vi "Push Border.vi"(8 "1D Maze":i32[](array[numeric]), 9 "Post":T1, 11 "Class":refnum<class "Pinwheel.lvclass">) -> (3 "Class":refnum<class "Pinwheel.lvclass">)   [LabVIEW 2015, in "Pinwheel.lvclass"]
uses:
  Pinwheel.lvclass
  Square/Square.lvclass
  Type Defs/Direction Enum.ctl
  Type Defs/SB Type Defs.lvlib
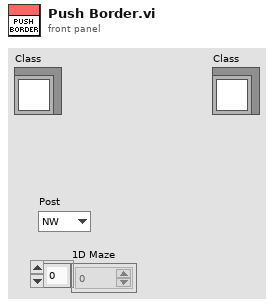
[diagram p1: front panel]
types:
  T1 = typedef "SB Type Defs.lvlib/Direction Enum.ctl" = enum16{"NW", "N", "NE", "E", "SE", "S", "SW", "W"}
  T2 = typedef "Pinwheel.lvclass/DVR Cluster.ctl" = cluster{"N":i32, "E":i32, "S":i32, "W":i32, "OD":T1, "NR":i32, "ER":i32, "SR":i32, "WR":i32, "NE":i32, "EE":i32, "SE":i32, "WE":i32, "Team":i32}
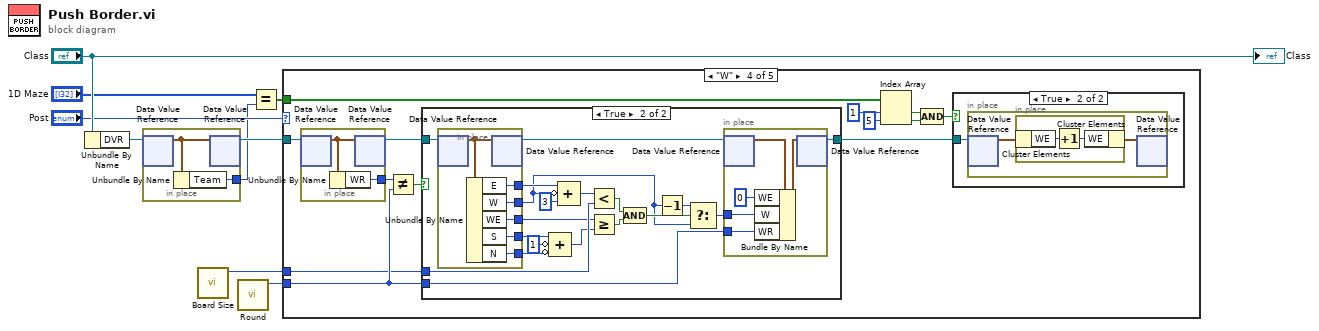
[diagram p0: block diagram]
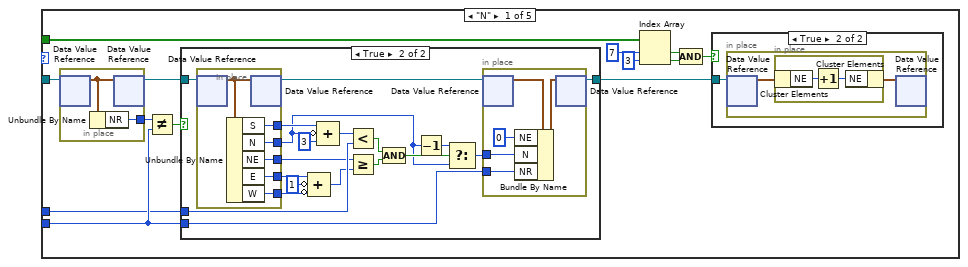
[diagram p2: hidden frame]
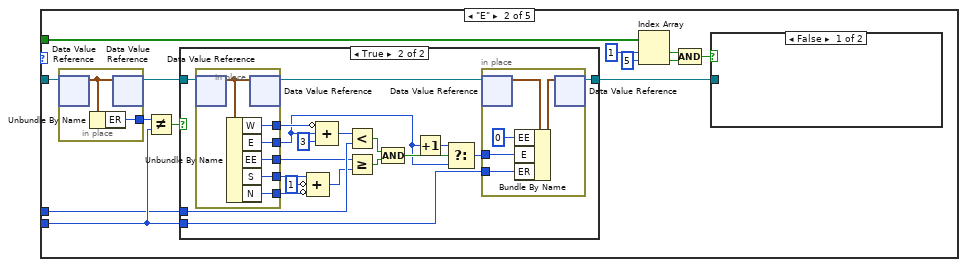
[diagram p5: hidden frame]
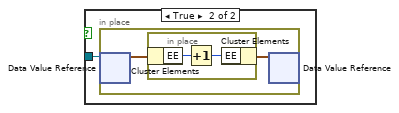
[diagram p7: hidden frame]
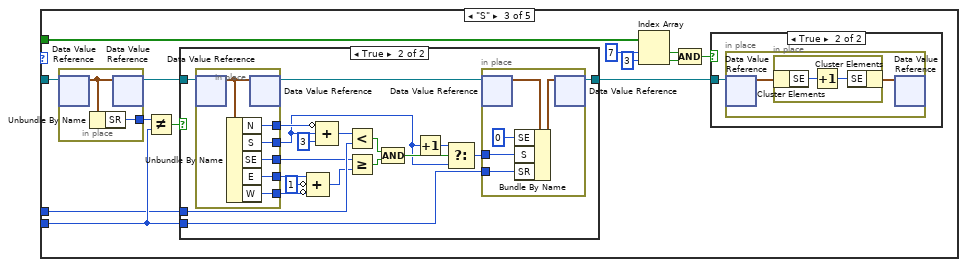
[diagram p8: hidden frame]
diagram:
  n1 = Unbundle By Name("Class") -> ("DVR"=w5:refnum<data-value>)
  n2 = in-place {
    in-place-border: [w10] -> w3
    n3 = in-place-dvr #1(w5) -> (w11:T2)  [unwired: 1 out]
    n4 = Unbundle By Name(w11) -> ("Team"=w10:i32)
    n5 = in-place-dvr #1(w11) -> (w4:refnum<data-value>)  [unwired: 1 out]
  }
  n6 = call "Board Size.vi"() -> ("Board Size"=w6:i32)  [unwired: 11 in]
  n7 = call "Round.vi"() -> ("Round"=w7:i32)  [unwired: 11 in]
  n8 = Equal?(x="1D Maze", y=w3) -> (x = y?=w1:bool[])
  n9 = case shown="\"W\"" "Post" {
    tunnel: w4 -> [w18 w69 w120 w171 _]
    tunnel: w1 -> [w24 w75 w126 w177 _]
    tunnel: w7 -> [w14 w65 w116 w167 _]
    tunnel: w6 -> [w13 w64 w115 w166 _]
    frame "N" {
      n10 = in-place {
        in-place-border: [w56] -> w17
        n11 = in-place-dvr #2(w18) -> (w57:T2)  [unwired: 1 out]
        n12 = Unbundle By Name(w57) -> ("NR"=w56:i32)
        n13 = in-place-dvr #2(w57) -> (w16:refnum<data-value>)  [unwired: 1 out]
      }
      n14 = Not Equal?(x=w17, y=w14) -> (x != y?=w15:bool)
      n15 = case shown="True" w15 {
        tunnel: w16 -> [w25 w43]
        tunnel: w14 -> [_ w44]
        tunnel: w13 -> [_ w37]
        tunnel: [w25 w32] -> w12
        frame False {
        }
        frame True {
          n16 = in-place {
            in-place-border: [w49] -> w28
            in-place-border: [w48] -> w34
            in-place-border: [w47] -> w40
            in-place-border: [w46] -> w31
            in-place-border: [w45] -> w30
            n17 = in-place-dvr #3(w43) -> (w50:T2)  [unwired: 1 out]
            n18 = Unbundle By Name(w50) -> ("S"=w47:i32, "N"=w48:i32, "NE"=w49:i32, "E"=w46:i32, "W"=w45:i32)
            n19 = in-place-dvr #3(w50) -> (w42:refnum<data-value>)  [unwired: 1 out]
          }
          n20 = Compound Arithmetic op=ADD(w31, invert 1 ("value"), invert w30) -> (w27:i32)
          n21 = Compound Arithmetic op=ADD(w40, invert w34, 3 ("value")) -> (w38:i32)
          n22 = Less?(x=w38, y=w37) -> (x < y?=w36:bool)
          n23 = Greater Or Equal?(x=w28, y=w27) -> (x >= y?=w29:bool)
          n24 = Compound Arithmetic op=AND(w36, w29) -> (w41:bool)
          n25 = Decrement(x=w34) -> (x-1=w35:i32)
          n26 = Select(t=w35, s=w41, f=w34) -> (s? t:f=w33:i32)
          n27 = in-place {
            in-place-border: w44 -> [w52]
            in-place-border: w33 -> [w53]
            n28 = in-place-dvr #4(w42) -> (w55:T2)  [unwired: 1 out]
            n29 = Bundle By Name(cluster=w55, "NE"=0, "N"=w53, "NR"=w52) -> (w54:T2)
            n30 = in-place-dvr #4(w54) -> (w32:refnum<data-value>)  [unwired: 1 out]
          }
        }
      }
      n31 = Index Array(array=w24, index #1=7 ("index"), index #2=3 ("index")) -> (element #1=w21:bool, element #2=w20:bool)
      n32 = Compound Arithmetic op=AND(w21, w20) -> (w19:bool)
      n33 = case shown="True" w19 {
        tunnel: w12 -> [_ w58]
        frame False {
        }
        frame True {
          n34 = in-place {
            n35 = in-place-dvr #5(w58) -> (w60:T2)  [unwired: 1 out]
            n36 = in-place {
              n37 = in-place-cluster #6(w60) -> ("NE"=w62:i32)
              n38 = Increment(x=w62) -> (x+1=w61:i32)
              n39 = in-place-cluster #6("NE"=w61) -> (w59:T2)
            }
            n40 = in-place-dvr #5(w59) -> ()  [unwired: 2 out]
          }
        }
      }
    }
    frame "E" {
      n41 = in-place {
        in-place-border: [w107] -> w68
        n42 = in-place-dvr #7(w69) -> (w108:T2)  [unwired: 1 out]
        n43 = Unbundle By Name(w108) -> ("ER"=w107:i32)
        n44 = in-place-dvr #7(w108) -> (w67:refnum<data-value>)  [unwired: 1 out]
      }
      n45 = Not Equal?(x=w68, y=w65) -> (x != y?=w66:bool)
      n46 = case shown="True" w66 {
        tunnel: w67 -> [w76 w94]
        tunnel: w65 -> [_ w95]
        tunnel: w64 -> [_ w88]
        tunnel: [w76 w83] -> w63
        frame False {
        }
        frame True {
          n47 = in-place {
            in-place-border: [w100] -> w79
            in-place-border: [w99] -> w85
            in-place-border: [w98] -> w91
            in-place-border: [w97] -> w82
            in-place-border: [w96] -> w81
            n48 = in-place-dvr #8(w94) -> (w101:T2)  [unwired: 1 out]
            n49 = Unbundle By Name(w101) -> ("W"=w98:i32, "E"=w99:i32, "EE"=w100:i32, "S"=w97:i32, "N"=w96:i32)
            n50 = in-place-dvr #8(w101) -> (w93:refnum<data-value>)  [unwired: 1 out]
          }
          n51 = Compound Arithmetic op=ADD(w82, invert 1 ("value"), invert w81) -> (w78:i32)
          n52 = Compound Arithmetic op=ADD(invert w91, w85, 3 ("value")) -> (w89:i32)
          n53 = Less?(x=w89, y=w88) -> (x < y?=w87:bool)
          n54 = Greater Or Equal?(x=w79, y=w78) -> (x >= y?=w80:bool)
          n55 = Compound Arithmetic op=AND(w87, w80) -> (w92:bool)
          n56 = Increment(x=w85) -> (x+1=w86:i32)
          n57 = Select(t=w86, s=w92, f=w85) -> (s? t:f=w84:i32)
          n58 = in-place {
            in-place-border: w95 -> [w103]
            in-place-border: w84 -> [w104]
            n59 = in-place-dvr #9(w93) -> (w106:T2)  [unwired: 1 out]
            n60 = Bundle By Name(cluster=w106, "EE"=0 ("NE"), "E"=w104, "ER"=w103) -> (w105:T2)
            n61 = in-place-dvr #9(w105) -> (w83:refnum<data-value>)  [unwired: 1 out]
          }
        }
      }
      n62 = Index Array(array=w75, index #1=1 ("index"), index #2=5 ("index")) -> (element #1=w72:bool, element #2=w71:bool)
      n63 = Compound Arithmetic op=AND(w72, w71) -> (w70:bool)
      n64 = case shown="False" w70 {
        tunnel: w63 -> [_ w109]
        frame False {
        }
        frame True {
          n65 = in-place {
            n66 = in-place-dvr #10(w109) -> (w111:T2)  [unwired: 1 out]
            n67 = in-place {
              n68 = in-place-cluster #11(w111) -> ("EE"=w113:i32)
              n69 = Increment(x=w113) -> (x+1=w112:i32)
              n70 = in-place-cluster #11("EE"=w112) -> (w110:T2)
            }
            n71 = in-place-dvr #10(w110) -> ()  [unwired: 2 out]
          }
        }
      }
    }
    frame "S" {
      n72 = in-place {
        in-place-border: [w158] -> w119
        n73 = in-place-dvr #12(w120) -> (w159:T2)  [unwired: 1 out]
        n74 = Unbundle By Name(w159) -> ("SR"=w158:i32)
        n75 = in-place-dvr #12(w159) -> (w118:refnum<data-value>)  [unwired: 1 out]
      }
      n76 = Not Equal?(x=w119, y=w116) -> (x != y?=w117:bool)
      n77 = case shown="True" w117 {
        tunnel: w118 -> [w127 w145]
        tunnel: w116 -> [_ w146]
        tunnel: w115 -> [_ w139]
        tunnel: [w127 w134] -> w114
        frame False {
        }
        frame True {
          n78 = in-place {
            in-place-border: [w151] -> w130
            in-place-border: [w150] -> w136
            in-place-border: [w149] -> w142
            in-place-border: [w148] -> w133
            in-place-border: [w147] -> w132
            n79 = in-place-dvr #13(w145) -> (w152:T2)  [unwired: 1 out]
            n80 = Unbundle By Name(w152) -> ("N"=w149:i32, "S"=w150:i32, "SE"=w151:i32, "E"=w148:i32, "W"=w147:i32)
            n81 = in-place-dvr #13(w152) -> (w144:refnum<data-value>)  [unwired: 1 out]
          }
          n82 = Compound Arithmetic op=ADD(w133, invert 1 ("value"), invert w132) -> (w129:i32)
          n83 = Compound Arithmetic op=ADD(invert w142, w136, 3 ("value")) -> (w140:i32)
          n84 = Less?(x=w140, y=w139) -> (x < y?=w138:bool)
          n85 = Greater Or Equal?(x=w130, y=w129) -> (x >= y?=w131:bool)
          n86 = Compound Arithmetic op=AND(w138, w131) -> (w143:bool)
          n87 = Increment(x=w136) -> (x+1=w137:i32)
          n88 = Select(t=w137, s=w143, f=w136) -> (s? t:f=w135:i32)
          n89 = in-place {
            in-place-border: w146 -> [w154]
            in-place-border: w135 -> [w155]
            n90 = in-place-dvr #14(w144) -> (w157:T2)  [unwired: 1 out]
            n91 = Bundle By Name(cluster=w157, "SE"=0 ("NE"), "S"=w155, "SR"=w154) -> (w156:T2)
            n92 = in-place-dvr #14(w156) -> (w134:refnum<data-value>)  [unwired: 1 out]
          }
        }
      }
      n93 = Index Array(array=w126, index #1=7 ("index"), index #2=3 ("index")) -> (element #1=w123:bool, element #2=w122:bool)
      n94 = Compound Arithmetic op=AND(w123, w122) -> (w121:bool)
      n95 = case shown="True" w121 {
        tunnel: w114 -> [_ w160]
        frame False {
        }
        frame True {
          n96 = in-place {
            n97 = in-place-dvr #15(w160) -> (w162:T2)  [unwired: 1 out]
            n98 = in-place {
              n99 = in-place-cluster #16(w162) -> ("SE"=w164:i32)
              n100 = Increment(x=w164) -> (x+1=w163:i32)
              n101 = in-place-cluster #16("SE"=w163) -> (w161:T2)
            }
            n102 = in-place-dvr #15(w161) -> ()  [unwired: 2 out]
          }
        }
      }
    }
    frame "W" {
      n103 = in-place {
        in-place-border: [w209] -> w170
        n104 = in-place-dvr #17(w171) -> (w210:T2)  [unwired: 1 out]
        n105 = Unbundle By Name(w210) -> ("WR"=w209:i32)
        n106 = in-place-dvr #17(w210) -> (w169:refnum<data-value>)  [unwired: 1 out]
      }
      n107 = Not Equal?(x=w170, y=w167) -> (x != y?=w168:bool)
      n108 = case shown="True" w168 {
        tunnel: w169 -> [w178 w196]
        tunnel: w167 -> [_ w197]
        tunnel: w166 -> [_ w190]
        tunnel: [w178 w185] -> w165
        frame False {
        }
        frame True {
          n109 = in-place {
            in-place-border: [w202] -> w181
            in-place-border: [w201] -> w187
            in-place-border: [w200] -> w193
            in-place-border: [w199] -> w184
            in-place-border: [w198] -> w183
            n110 = in-place-dvr #18(w196) -> (w203:T2)  [unwired: 1 out]
            n111 = Unbundle By Name(w203) -> ("E"=w200:i32, "W"=w201:i32, "WE"=w202:i32, "S"=w199:i32, "N"=w198:i32)
            n112 = in-place-dvr #18(w203) -> (w195:refnum<data-value>)  [unwired: 1 out]
          }
          n113 = Compound Arithmetic op=ADD(w184, invert 1 ("value"), invert w183) -> (w180:i32)
          n114 = Compound Arithmetic op=ADD(w193, invert w187, 3 ("value")) -> (w191:i32)
          n115 = Less?(x=w191, y=w190) -> (x < y?=w189:bool)
          n116 = Greater Or Equal?(x=w181, y=w180) -> (x >= y?=w182:bool)
          n117 = Compound Arithmetic op=AND(w189, w182) -> (w194:bool)
          n118 = Decrement(x=w187) -> (x-1=w188:i32)
          n119 = Select(t=w188, s=w194, f=w187) -> (s? t:f=w186:i32)
          n120 = in-place {
            in-place-border: w197 -> [w205]
            in-place-border: w186 -> [w206]
            n121 = in-place-dvr #19(w195) -> (w208:T2)  [unwired: 1 out]
            n122 = Bundle By Name(cluster=w208, "WE"=0 ("NE"), "W"=w206, "WR"=w205) -> (w207:T2)
            n123 = in-place-dvr #19(w207) -> (w185:refnum<data-value>)  [unwired: 1 out]
          }
        }
      }
      n124 = Index Array(array=w177, index #1=1 ("index"), index #2=5 ("index")) -> (element #1=w174:bool, element #2=w173:bool)
      n125 = Compound Arithmetic op=AND(w174, w173) -> (w172:bool)
      n126 = case shown="True" w172 {
        tunnel: w165 -> [_ w211]
        frame False {
        }
        frame True {
          n127 = in-place {
            n128 = in-place-dvr #20(w211) -> (w213:T2)  [unwired: 1 out]
            n129 = in-place {
              n130 = in-place-cluster #21(w213) -> ("WE"=w215:i32)
              n131 = Increment(x=w215) -> (x+1=w214:i32)
              n132 = in-place-cluster #21("WE"=w214) -> (w212:T2)
            }
            n133 = in-place-dvr #20(w212) -> ()  [unwired: 2 out]
          }
        }
      }
    }
    frame Default {
    }
  }
  "Class" <- "Class"
